vi "Initiate Traverse System.vi"(8 "error in":errorcluster, 10 "VISA resource name":refnum<visa-resource-name>, 11 "Water Tunnel Results in":refnum<class "Water Tunnel Results.lvclass">) -> (0 "error out":errorcluster, 3 "Water Tunnel Results out":refnum<class "Water Tunnel Results.lvclass">)   [LabVIEW 2019, in "Results.lvlib" / "Water Tunnel Results.lvclass"]
uses:
  Water Tunnel Results.lvclass
panel:
  out "read buffer":string
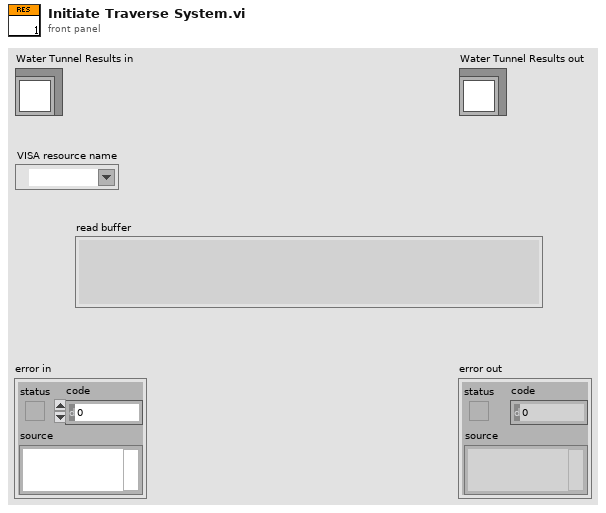
[diagram p1: front panel]
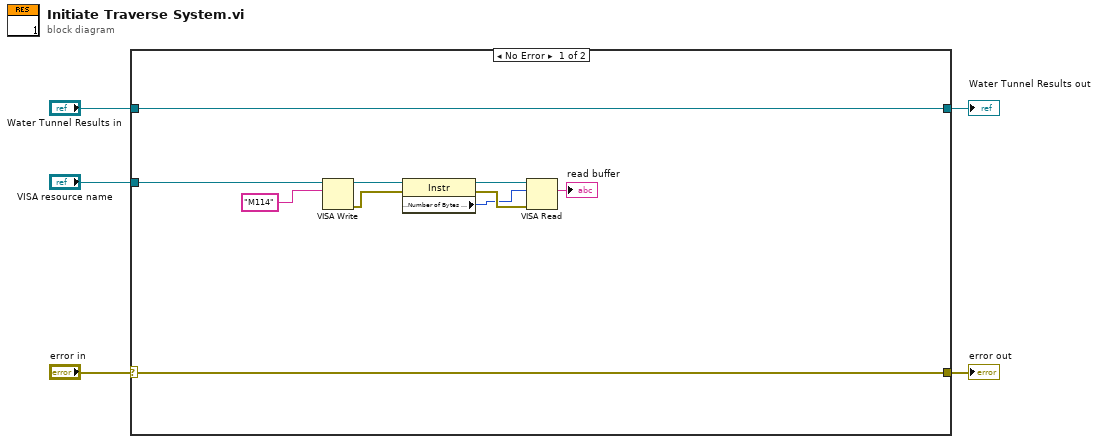
[diagram p0: block diagram]
diagram:
  n1 = case shown="No Error" "error in" {
    selector: "error in" -> [w14 w17]
    tunnel: [w14 w17] -> w4
    tunnel: [w15 w16] -> w2
    tunnel: "Water Tunnel Results in" -> [w15 w16]
    tunnel: "VISA resource name" -> [w13 _]
    frame No Error {
      n2 = VISA Write(VISA resource name=w13, write buffer="M114") -> (VISA resource name out=w12:refnum<visa-resource-name>, error out=w10:errorcluster)  [unwired: 1 in, 1 out]
      n3 = property class="Instr"(reference=w12, error in=w10) -> (reference out=w11:refnum<visa-resource-name>, error out=w9:errorcluster, "Serial Settings:Number of Bytes at Serial Port"=w8:u32)
      n4 = VISA Read(VISA resource name=w11, byte count=w8, error in (no error)=w9) -> (read buffer=→"read buffer":string)  [unwired: 3 out]
    }
    frame Error {
    }
  }
  "error out" <- w4
  "Water Tunnel Results out" <- w2
